vi "ClearExcelData.vi"(8 "error in (no error)":errorcluster, 11 "Path":path) -> ()   [LabVIEW 2020]
panel:
  in  "Excel._Worksheet 2":refnum<k7>
  in  "Excel._Worksheet":refnum<k7>
  in  "Excel._Application":refnum<k7>
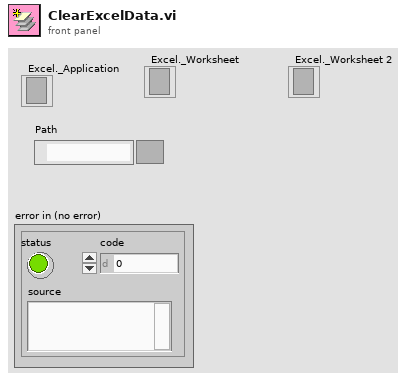
[diagram p1: front panel]
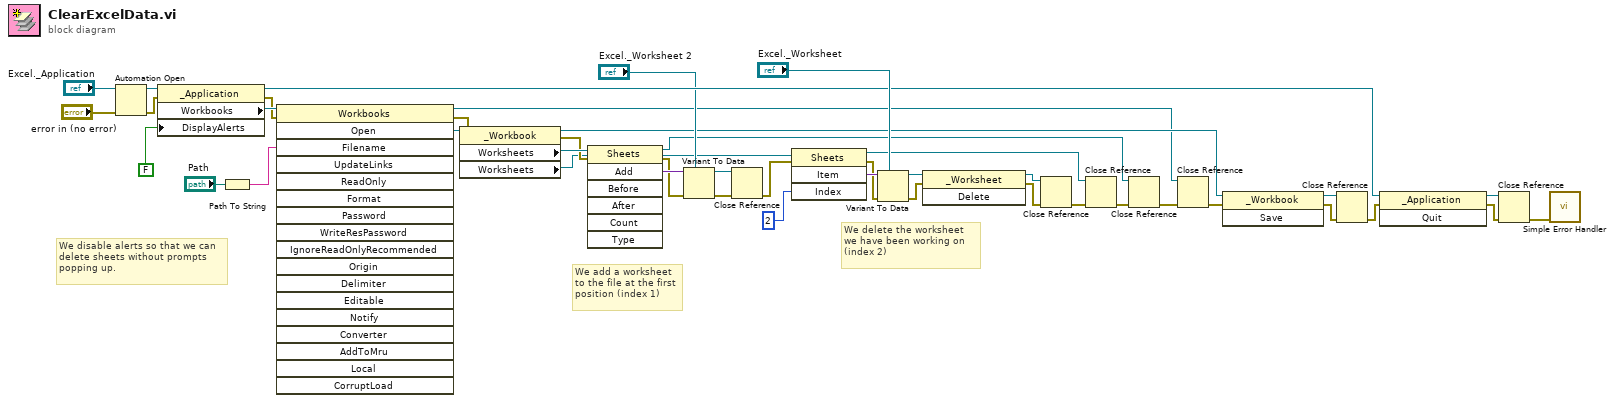
[diagram p0: block diagram]
diagram:
  # "We delete the worksheet\nwe have been working on\n(index 2)"
  # "We add a worksheet\nto the file at the first\nposition (index 1)"
  # "We disable alerts so that we can\ndelete sheets without prompts\npopping up."
  n1 = Automation Open(error in (no error)="error in (no error)", Automation Refnum="Excel._Application") -> (Automation Refnum=w42:refnum<k7>, error out=w34:errorcluster)  [unwired: 2 in]
  n2 = property class="_Application"(reference=w42, error in=w34, "DisplayAlerts"=FALSE ("Visible")) -> (reference out=w37:refnum<k7>, error out=w33:errorcluster, "Workbooks"=w41:refnum<k7>)
  n3 = Path To String(path="Path") -> (string=w38:string)
  n4 = invoke class="Workbooks" method="Open"(reference=w41, error in=w33, "Filename"=w38) -> (reference out=w8:refnum<k7>, error out=w31:errorcluster, "Open"=w22:refnum<k7>)  [unwired: 15 in, 15 out]
  n5 = property class="_Workbook"(reference=w22, error in=w31) -> (reference out=w21:refnum<k7>, error out=w29:errorcluster, "Worksheets"=w30:refnum<k7>, "Worksheets"=w7:refnum<k7>)
  n6 = invoke class="Sheets" method="Add"(reference=w30, error in=w29) -> (reference out=w4:refnum<k7>, error out=w27:errorcluster, "Add"=w28:variant)  [unwired: 5 in, 4 out]
  n7 = Variant To Data(error in=w27, type="Excel._Worksheet 2", Variant=w28) -> (data=w25:refnum<k7>, error out=w24:errorcluster)
  n8 = Close Reference(reference=w25, error in (no error)=w24) -> (error out=w23:errorcluster)
  n9 = invoke class="Sheets" method="Item"(reference=w7, error in=w23, "Index"=2) -> (reference out=w12:refnum<k7>, error out=w18:errorcluster, "Item"=w19:variant)  [unwired: 1 in, 1 out]
  n10 = Variant To Data(error in=w18, type="Excel._Worksheet", Variant=w19) -> (data=w17:refnum<k7>, error out=w16:errorcluster)
  n11 = invoke class="_Worksheet" method="Delete"(reference=w17, error in=w16) -> (reference out=w15:refnum<k7>, error out=w14:errorcluster)  [unwired: 1 in, 1 out]
  n12 = Close Reference(reference=w15, error in (no error)=w14) -> (error out=w13:errorcluster)
  n13 = Close Reference(reference=w12, error in (no error)=w13) -> (error out=w6:errorcluster)
  n14 = Close Reference(reference=w4, error in (no error)=w6) -> (error out=w5:errorcluster)
  n15 = Close Reference(reference=w8, error in (no error)=w5) -> (error out=w9:errorcluster)
  n16 = invoke class="_Workbook" method="Save"(reference=w21, error in=w9) -> (reference out=w2:refnum<k7>, error out=w3:errorcluster)  [unwired: 1 in, 1 out]
  n17 = Close Reference(reference=w2, error in (no error)=w3) -> (error out=w1:errorcluster)
  n18 = invoke class="_Application" method="Quit"(reference=w37, error in=w1) -> (reference out=w36:refnum<k7>, error out=w32:errorcluster)  [unwired: 1 in, 1 out]
  n19 = Close Reference(reference=w36, error in (no error)=w32) -> (error out=w10:errorcluster)
  n20 = call <vilib>:"Simple Error Handler.vi"("error in (no error)"=w10) -> ()  [unwired: 4 in, 5 out]
